vi "binary_to_dec.vi"() -> ()   [LabVIEW 2026]
panel:
  out "DECIMAL":dbl
  in  "BIT 1:LSB_RIGHT":bool
  in  "BIT 2":bool
  in  "BIT 3":bool
  in  "BIT 4: MSB_LEFT":bool
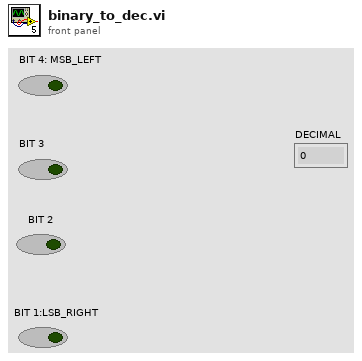
[diagram p1: front panel]
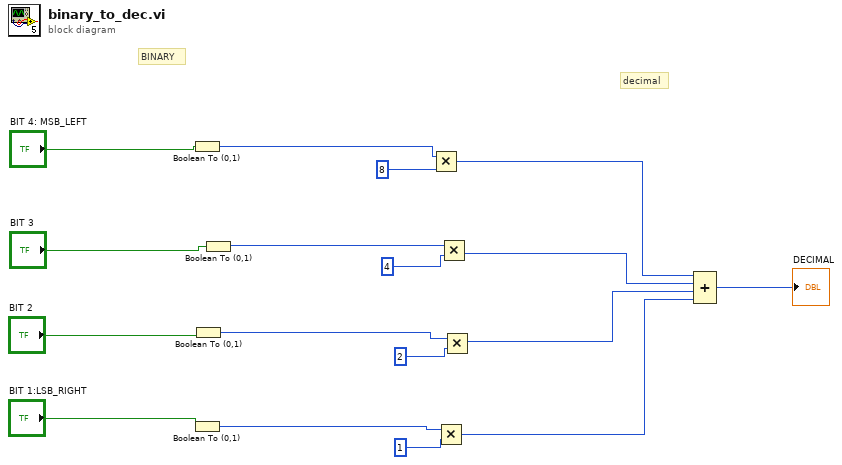
[diagram p0: block diagram]
diagram:
  # "decimal"
  # "BINARY"
  n1 = Boolean To (0,1)(Boolean="BIT 4: MSB_LEFT") -> (0, 1=w13:i16)
  n2 = Boolean To (0,1)(Boolean="BIT 1:LSB_RIGHT") -> (0, 1=w10:i16)
  n3 = Boolean To (0,1)(Boolean="BIT 2") -> (0, 1=w11:i16)
  n4 = Boolean To (0,1)(Boolean="BIT 3") -> (0, 1=w12:i16)
  n5 = Multiply(x=w13, y=8) -> (x*y=w5:i32)
  n6 = Multiply(x=w10, y=1) -> (x*y=w2:i32)
  n7 = Multiply(x=w12, y=4) -> (x*y=w4:i32)
  n8 = Multiply(x=w11, y=2) -> (x*y=w3:i32)
  n9 = Compound Arithmetic op=ADD(w5, w4, w3, w2) -> (→"DECIMAL":i32)
